vi "Live window-Event handler-distance locked.vi"(11 "Function":T1) -> ()   [LabVIEW 2013]
uses:
  Typedefs/Left-Right enum.ctl
  Globals/gl_Windows Ctrl refs.vi
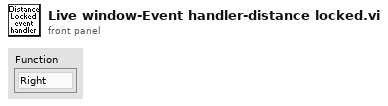
[diagram p1: front panel]
types:
  T1 = typedef "Left-Right enum.ctl" = enum16{"Right", "Left"}
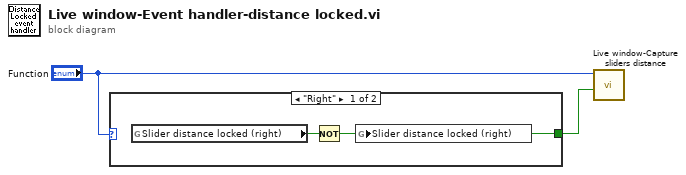
[diagram p0: block diagram]
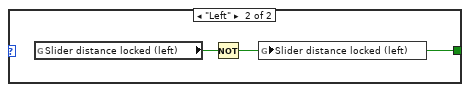
[diagram p2: hidden frame]
diagram:
  n1 = case shown="\"Right\"" "Function" {
    tunnel: [w3 w5] -> w2
    frame "Right" {
      n2 = global read "gl_Windows Ctrl refs.vi" "Slider distance locked (right)"() -> (w4:bool)
      n3 = Not(x=w4) -> (.not. x?=w3:bool)
      n4 = global write "gl_Windows Ctrl refs.vi" "Slider distance locked (right)"(w3) -> ()
    }
    frame "Left" {
      n5 = global read "gl_Windows Ctrl refs.vi" "Slider distance locked (left)"() -> (w6:bool)
      n6 = Not(x=w6) -> (.not. x?=w5:bool)
      n7 = global write "gl_Windows Ctrl refs.vi" "Slider distance locked (left)"(w5) -> ()
    }
  }
  n8 = call "Live window-Capture sliders distance.vi"("Locked?"=w2, "Function"="Function") -> ()  [unwired: 10 in]
